vi "PID sensor w reset.vi"(4 "State":i16, 5 "Time":dbl format="%.2f", 6 "Sensor Values":dbl[](array[numeric]), 7 "Set Points":dbl[](array[numeric])) -> (0 "required data":T1={"Set Point names"=["target value", "P Kc", "I Ti (s)", "D Td (s)"], "required number of setpoints"=4, "required number of sensors"=1, "Sensor names"=["Measured process value"]}, 3 "output value":dbl)   [LabVIEW 2019]
uses:
  <vilib>/addons/control/pid/pid.llb/PID (DBL).vi
  <vilib>/addons/control/pid/NI_PID_pid.lvlib
panel:
  # "Enter the correct information for this control code in the required data structure below. Then make the current value default by right clicking on the border of the data structure."
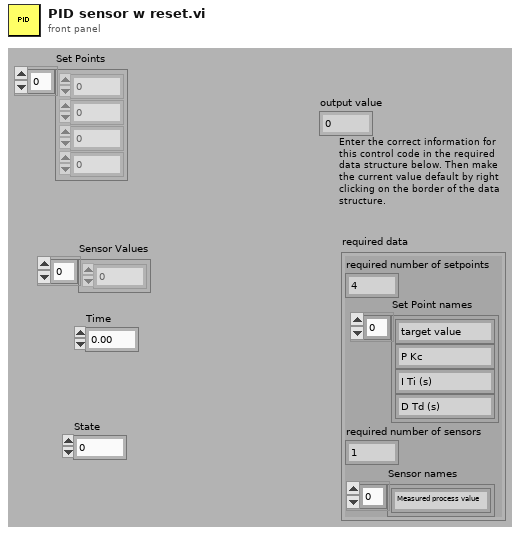
[diagram p1: front panel]
types:
  T1 = cluster{"Set Point names":string[], "required number of setpoints":u8, "required number of sensors":u8, "Sensor names":string[]}
  T2 = cluster{"Set Points[0]":dbl, "Set Points[1]":dbl, "Set Points[2]":dbl, "Set Points[3]":dbl}
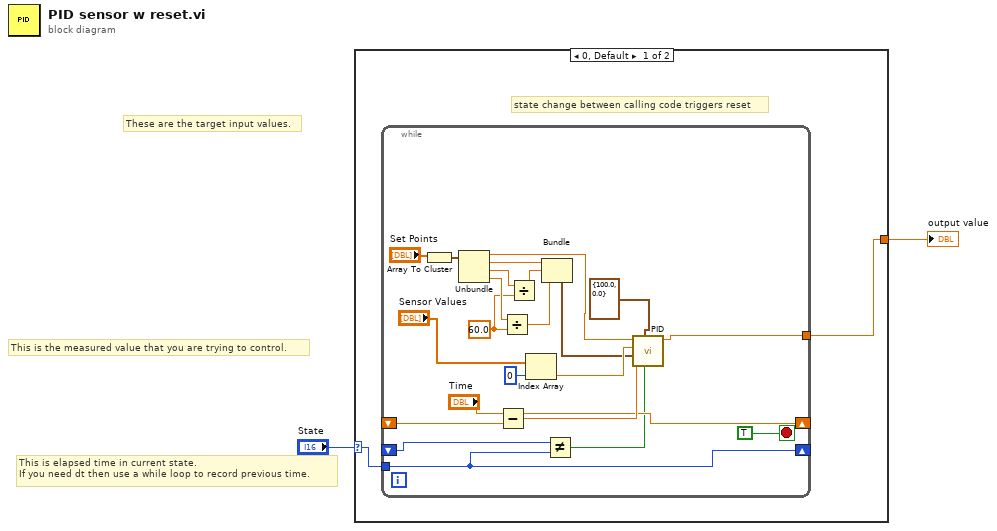
[diagram p0: block diagram]
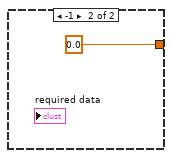
[diagram p2: hidden frame]
diagram:
  # "These are the target input values."
  # "This is the measured value that you are trying to control."
  # "This is elapsed time in current state.\nIf you need dt then use a while loop to record previous time."
  n1 = case shown="0, Default" "State" {
    selector: "State" -> [w3 _]
    tunnel: [w4 0.0 ("fraction on")] -> w2
    frame 0, Default {
      # "state change between calling code triggers reset"
      n2 = while {
        shift-right: ["Time"] -> _
        shift-left: _ -> [w25]
        tunnel: [w10] -> w4
        shift-right: [w14] -> _
        shift-left: _ -> [w15]
        tunnel: w3 -> [w14]
        stop <- TRUE stop-if-true
        w6 = 60.0 ("y")
        n3 = Array To Cluster(array="Set Points") -> (cluster=w21:T2)
        n4 = Unbundle(w21) -> ("Set Points[0]"=w16:dbl, "Set Points[1]"=w20:dbl, "Set Points[2]"=w7:dbl, "Set Points[3]"=w9:dbl)
        n5 = Subtract(x="Time", y=w25) -> (x-y=w24:dbl)
        n6 = Divide(x=w9, y=w6) -> (x/y=w8:dbl)
        n7 = Divide(x=w7, y=w6) -> (x/y=w5:dbl)
        n8 = Index Array(array="Sensor Values", index=0) -> (element=w17:dbl)
        n9 = Bundle("Set Points[1]"=w20, w5, w8) -> (w12:cluster{"Set Points[1]":dbl, dbl, dbl})  [unwired: 1 in]
        n10 = Not Equal?(x=w15, y=w14) -> (x != y?=w13:bool)
        n11 = call-poly <vilib>:"PID.vi"("reinitialize? (F)"=w13, "output range"=cluster{"output high":dbl, "output low":dbl} {"output high"=100.0, "output low"=0.0}, "dt (s)"=w24, "PID gains"=w12, "process variable"=w17, "setpoint"=w16) -> ("output"=w10:dbl)  [unwired: 4 in, 1 out]
      }
    }
    frame -1 {
    }
  }
  "output value" <- w2
